vi "WPI_DigitalModuleSetPWMPeriodScale.vi"(8 "error in (no error)":errorcluster, 9 "PeriodScale":u8, 10 "PWMChannel":T1=enum."PWM 1") -> (0 "error out":errorcluster)   [LabVIEW 2017]
doc: "This software is licensed. Open the labview\\readme\\WPI Robotics Library Open Source License.txt file for more information."
uses:
  <vilib>/Rock Robotics/SystemInterfaces/DIO/FPGA_DIOPWMChannel.ctl
  <vilib>/Rock Robotics/SystemInterfaces/System/FPGA_SystemGet.vi
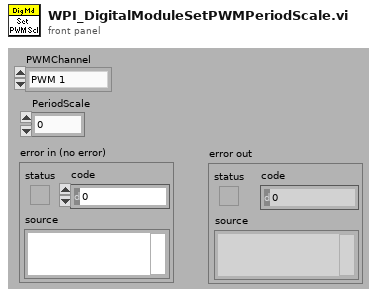
[diagram p1: front panel]
types:
  T1 = typedef "FPGA_DIOPWMChannel.ctl" = enum8{"PWM 0", "PWM 1", "PWM 2", "PWM 3", "PWM 4", "PWM 5", "PWM 6", "PWM 7", "PWM 8", "PWM 9", "PWM MXP 0", "PWM MXP 1", "PWM MXP 2", "PWM MXP 3", "PWM MXP 4", "PWM MXP 5", "PWM MXP 6", "PWM MXP 7", "PWM MXP 8", "PWM MXP 9", "Invalid"}
  T2 = typedef "FPGA_DIODevRef.ctl" = cluster{"DevStatus":errorcluster}
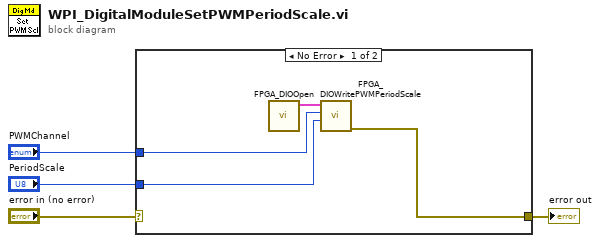
[diagram p0: block diagram]
diagram:
  n1 = case shown="No Error" "error in (no error)" {
    selector: "error in (no error)" -> [_ w9]
    tunnel: [w5 w9] -> w3
    tunnel: "PeriodScale" -> [w6 _]
    tunnel: "PWMChannel" -> [w7 _]
    frame No Error {
      n2 = call <vilib>:"FPGA_DIOOpen.vi"() -> ("DIODeviceRef"=w8:T2)  [unwired: 2 in, 9 out]
      n3 = call <vilib>:"FPGA_DIOWritePWMPeriodScale.vi"("PWMPeriodScale"=w6, "PWMChannel"=w7, "DIODeviceRef In"=w8) -> ("error out"=w5:errorcluster)  [unwired: 1 in, 7 out]
    }
    frame Error {
    }
  }
  "error out" <- w3
